vi "Set Series Base.lvclass.vi"(8 "error in (no error)":errorcluster, 10 "HAL GOOP4.lvlib:Study Base.lvclass":refnum<class "Series Base.lvclass">, 11 "Series Actor in":refnum<class "Series Actor.lvclass">) -> (0 "error out":errorcluster, 3 "Series Actor out":refnum<class "Series Actor.lvclass">)   [LabVIEW 2023, in "Series Actor.lvlib" / "Series Actor.lvclass"]
uses:
  Series Actor.lvclass
  Series Base/Series Base.lvclass
  Series Actor.lvclass/Series Actor.ctl
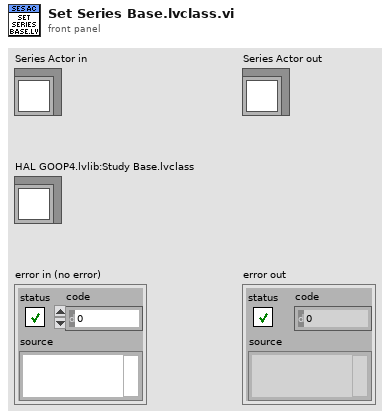
[diagram p1: front panel]
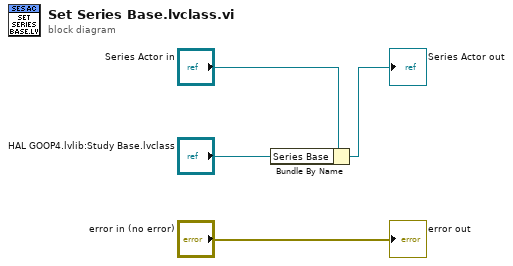
[diagram p0: block diagram]
diagram:
  n1 = Bundle By Name(cluster="Series Actor in", "Series Base"="HAL GOOP4.lvlib:Study Base.lvclass") -> (→"Series Actor out":refnum<class "Series Actor.lvclass">)
  "error out" <- "error in (no error)"
